vi "_API_BINANCE_GET_Getall.vi"(0 "BinanceAPI in":refnum<class "BinanceAPI_.lvclass">, 5 "GetAll":cluster{"recvWindow":string}={"recvWindow"="5000"}, 11 "error in (no error)":errorcluster) -> (4 "BinanceAPI out":refnum<class "BinanceAPI_.lvclass">, 6 "Data out":T1(array[cluster]), 14 "Data":string, 15 "error out":errorcluster)   [LabVIEW 2022 SP3, in "BinanceAPI_.lvclass"]
doc: "https://binance-docs.github.io/apidocs/spot/en/#all-coins-39-information-user_data"
uses:
  BinanceAPI_.lvclass
  BinanceAPI_.lvclass/BinanceAPI_.ctl
  783ded27-3ad3-4d15-b1f3-de020588183e.vi
  <vilib>/JDP Science/JSONtext/JSON text to Variant.vi
  <vilib>/JDP Science/JSONtext/LVClass Serializer/JSONtext LVClass Serializer.lvclass
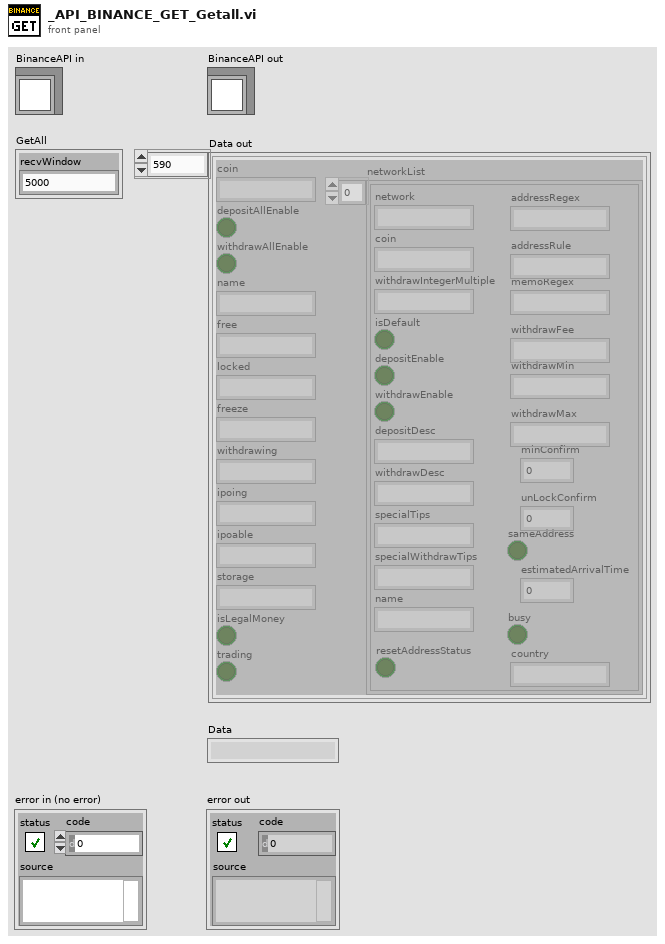
[diagram p1: front panel]
types:
  T1 = cluster{"coin":string, "depositAllEnable":bool, "withdrawAllEnable":bool, "name":string, "free":string, "locked":string, "freeze":string, "withdrawing":string, "ipoing":string, "ipoable":string, "storage":string, "isLegalMoney":bool, "trading":bool, "networkList":cluster{"network":string, "coin":string, "withdrawIntegerMultiple":string, "isDefault":bool, "depositEnable":bool, "withdrawEnable":bool, "depositDesc":string, "withdrawDesc":string, "specialTips":string, "specialWithdrawTips":string, "name":string, "resetAddressStatus":bool, "addressRegex":string, "addressRule":string, "memoRegex":string, "withdrawFee":string, "withdrawMin":string, "withdrawMax":string, "minConfirm":dbl, "unLockConfirm":dbl, "sameAddress":bool, "estimatedArrivalTime":dbl, "busy":bool, "country":string}[]}[]
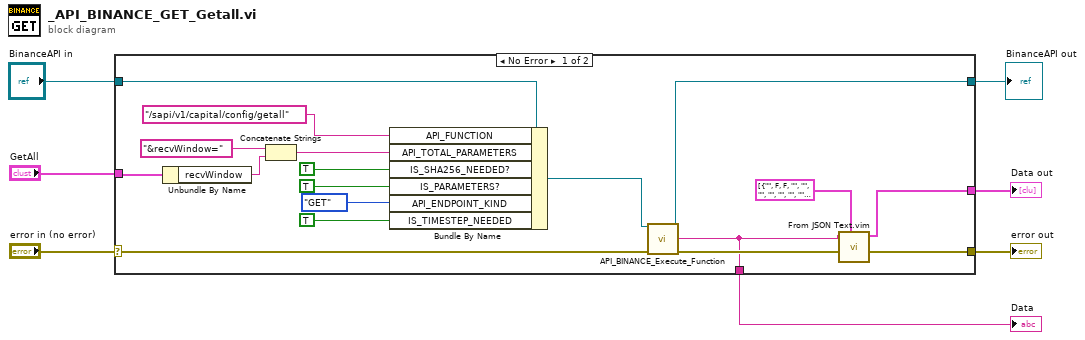
[diagram p0: block diagram]
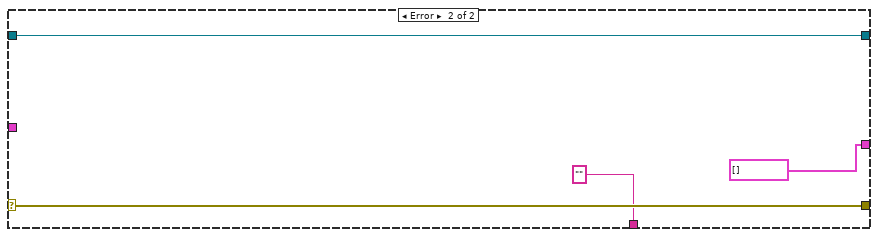
[diagram p2: hidden frame]
diagram:
  n1 = case shown="No Error" "error in (no error)" {
    selector: "error in (no error)" -> [w15 w29]
    tunnel: [w11 w29] -> w6
    tunnel: [w16 w26] -> w1
    tunnel: "GetAll" -> [w20 _]
    tunnel: [w8 "" ("Dane")] -> w4
    tunnel: [w13 T1 [] ("Data out")] -> w3
    tunnel: "BinanceAPI in" -> [w10 w26]
    frame No Error {
      n2 = Unbundle By Name(w20) -> ("recvWindow"=w22:string)
      n3 = Concatenate Strings("&recvWindow=" ("API_FUNCTION 2"), w22) -> (w21:string)
      n4 = Bundle By Name(cluster=w10, "API_FUNCTION"="/sapi/v1/capital/config/getall", "API_TOTAL_PARAMETERS"=w21, "IS_SHA256_NEEDED?"=TRUE, "IS_PARAMETERS?"=TRUE, "API_ENDPOINT_KIND"=enum16{"POST", "DELETE", "GET", "PUT"}."GET", "IS_TIMESTEP_NEEDED"=TRUE) -> (w9:refnum<class "BinanceAPI_.lvclass">)
      n5 = call "API_BINANCE_Execute_Function.vi"("BinanceAPI in"=w9, "error in (no error)"=w15) -> ("BinanceAPI out"=w16:refnum<class "BinanceAPI_.lvclass">, "Body"=w8:string, "error out"=w12:errorcluster)  [unwired: 9 in, 2 out]
      n6 = call "From JSON Text.vim"("Data Type and Default Value"=T1 [{"coin"="", "depositAllEnable"=FALSE, "withdrawAllEnable"=FALSE, "name"="", "free"="", "locked"="", "freeze"="", "withdrawing"="", "ipoing"="", "ipoable"="", "storage"="", "isLegalMoney"=FALSE, "trading"=FALSE, "networkList"=[{"network"="", "coin"="", "withdrawIntegerMultiple"="", "isDefault"=FALSE, "depositEnable"=FALSE, "withdrawEnable"=FALSE, "depositDesc"="", "withdrawDesc"="", "specialTips"="", "specialWithdrawTips"="", "name"="", "resetAddressStatus"=FALSE, "addressRegex"="", "addressRule"="", "memoRegex"="", "withdrawFee"="", "withdrawMin"="", "withdrawMax"="", "minConfirm"=0.0, "unLockConfirm"=0.0, "sameAddress"=FALSE, "estimatedArrivalTime"=0.0, "busy"=FALSE, "country"=""}]}], "error in (no error)"=w12, "JSON"=w8) -> ("error out"=w11:errorcluster, "Data out"=w13:T1)  [unwired: 7 in]
    }
    frame Error {
    }
  }
  "error out" <- w6
  "Data" <- w4
  "Data out" <- w3
  "BinanceAPI out" <- w1
